vi "Data Acq Text Out.vi"(1 "Data Acq":T2={"New/Stop File"=enum."New File", "Comments Option"=FALSE, "Comments"="", "extra wait"=1} {"extra wait" min=0}) -> (0 "Command text":string[][](array[string]))   [LabVIEW 2024]
uses:
  Data Acq.ctl
panel:
  out "New/Stop File":T1(ring)
  out "String Cluster":T3
  # "AND wait extra"
  # "seconds"
  # "Advanced Control"
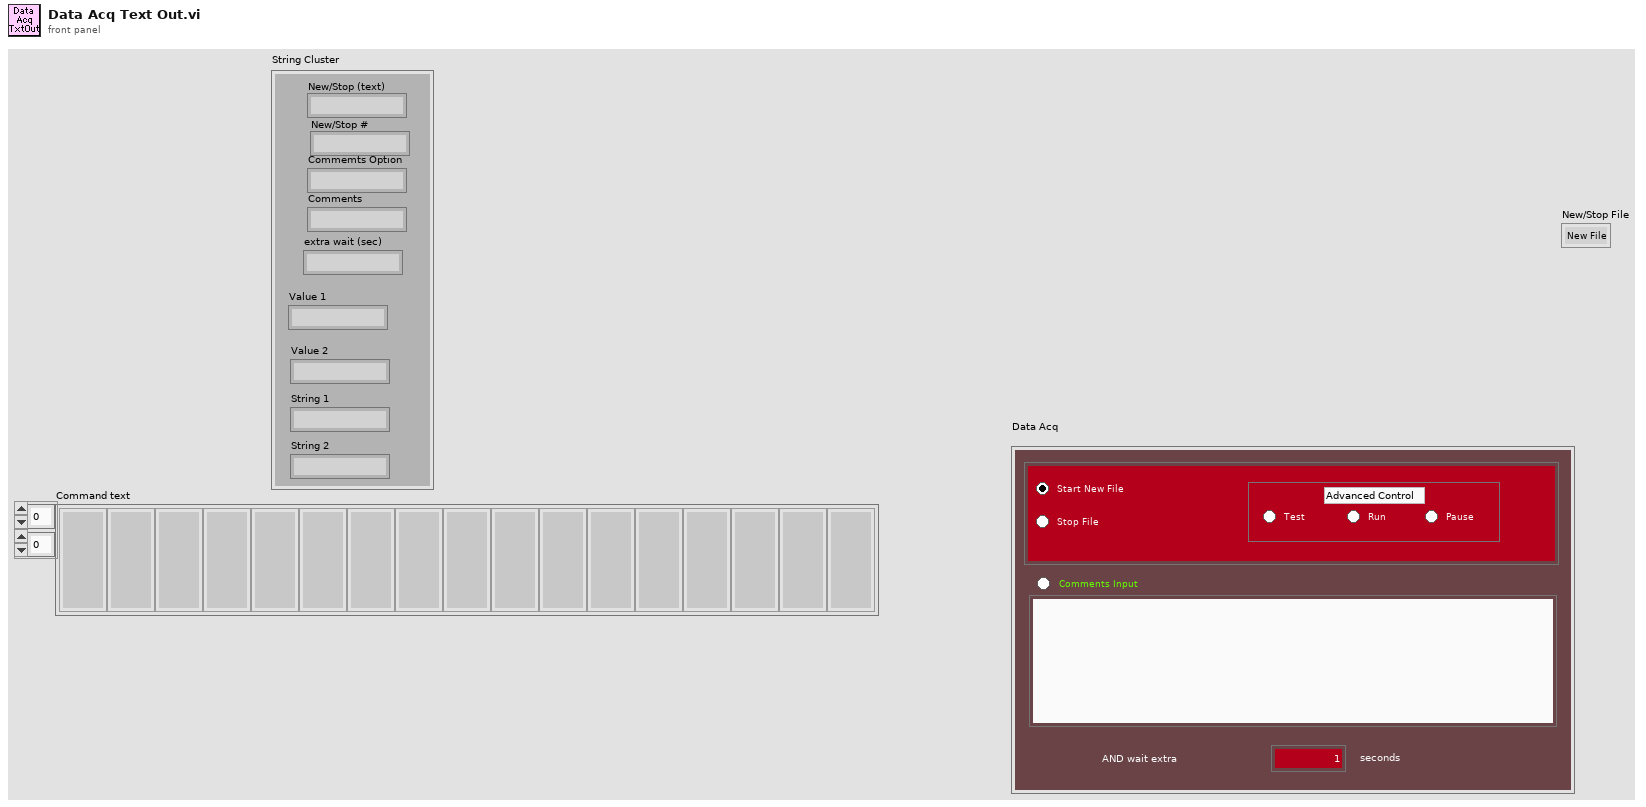
[diagram p1: front panel]
types:
  T1 = enum32{"New File", "Stop FIle", "Test", "Run", "Pause"}
  T2 = typedef "Data Acq.ctl" = cluster{"New/Stop File":enum32{"New File", "Stop FIle", "Test", "Run", "Pause"}, "Comments Option":bool, "Comments":string, "extra wait":i32}
  T3 = cluster{"New/Stop (text)":string, "Commemts Option":string, "Comments":string, "extra wait (sec)":string, "New/Stop #":string, "Value 1":string, "Value 2":string, "String 1":string, "String 2":string}
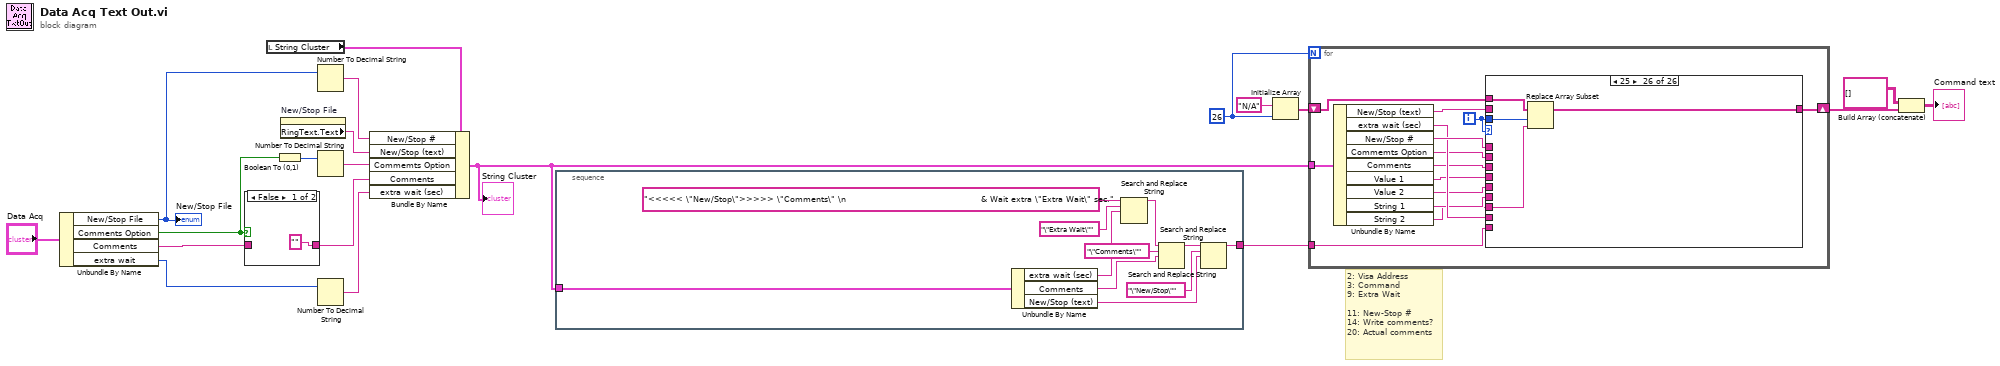
[diagram p0: block diagram]
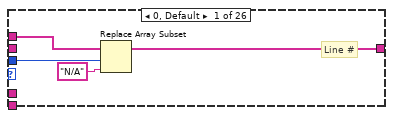
[diagram p3: hidden frame]
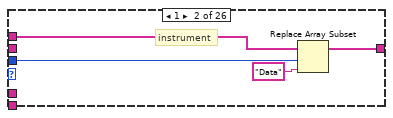
[diagram p4: hidden frame]
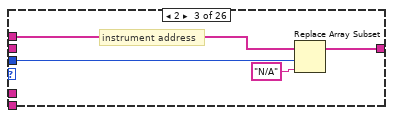
[diagram p5: hidden frame]
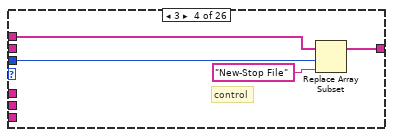
[diagram p6: hidden frame]
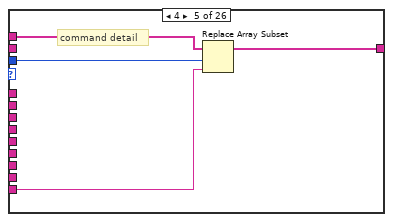
[diagram p7: hidden frame]
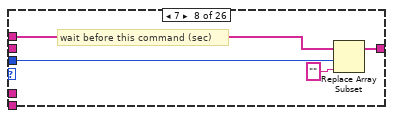
[diagram p10: hidden frame]
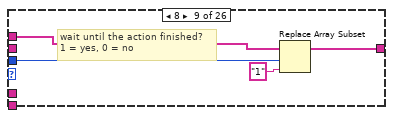
[diagram p11: hidden frame]
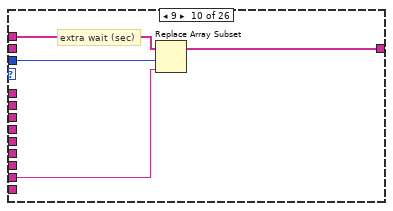
[diagram p12: hidden frame]
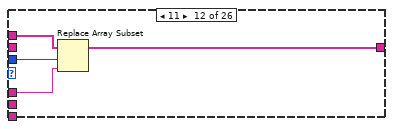
[diagram p14: hidden frame]
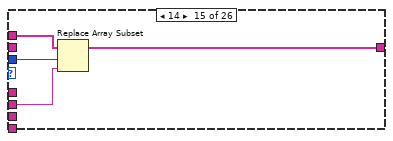
[diagram p17: hidden frame]
diagram:
  w17 = 26
  # "2: Visa Address\n3: Command\n9: Extra Wait\n\n11: New-Stop #\n14: Write comments?\n20: Actual comments"
  n1 = Unbundle By Name("Data Acq") -> ("New/Stop File"=w4:T1, "Comments Option"=w7:bool, "Comments"=w9:string, "extra wait"=w2:i32)
  "New/Stop File" <- w4
  n2 = case shown="False" w7 {
    tunnel: w9 -> [_ w22]
    tunnel: ["" w22] -> w8
    frame False {
    }
    frame True {
    }
  }
  n3 = local read "String Cluster"() -> (w14:T3)
  n4 = Boolean To (0,1)(Boolean=w7) -> (0, 1=w6:i16)
  n5 = property on="New/Stop File" class="Enum (strict)"() -> ("RingText.Text"=w10:string)  [unwired: 2 in, 2 out]
  n6 = Number To Decimal String(number=w4) -> (decimal integer string=w3:string)  [unwired: 1 in]
  n7 = Number To Decimal String(number=w6) -> (decimal integer string=w5:string)  [unwired: 1 in]
  n8 = Number To Decimal String(number=w2) -> (decimal integer string=w1:string)  [unwired: 1 in]
  n9 = Bundle By Name(cluster=w14, "New/Stop #"=w3, "New/Stop (text)"=w10, "Commemts Option"=w5, "Comments"=w8, "extra wait (sec)"=w1) -> (w12:T3)
  "String Cluster" <- w12
  n10 = stacked-sequence {
    tunnel: [w23] -> w13
    tunnel: w12 -> [w27]
    frame #0 {
      n11 = Unbundle By Name(w27) -> ("extra wait (sec)"=w26:string, "Comments"=w25:string, "New/Stop (text)"=w24:string)
      n12 = Search and Replace String(input string="<<<<< \"New/Stop\">>>>> \"Comments\" \n                                             & Wait extra \"Extra Wait\" sec.", search string="\"Extra Wait\"", replace string=w26) -> (result string=w32:string)  [unwired: 5 in, 3 out]
      n13 = Search and Replace String(input string=w32, search string="\"Comments\"", replace string=w25) -> (result string=w33:string)  [unwired: 5 in, 3 out]
      n14 = Search and Replace String(input string=w33, search string="\"New/Stop\"", replace string=w24) -> (result string=w23:string)  [unwired: 5 in, 3 out]
    }
  }
  n15 = Initialize Array("N/A", w17) -> (w16:string[])
  n16 = for {
    N: w17 -> [_]
    shift-right: [w45] -> w15
    shift-left: w16 -> [w46]
    tunnel: w13 -> [w44]
    tunnel: w12 -> [w43]
    i -> [w47]
    n17 = Unbundle By Name(w43) -> ("New/Stop (text)"=w41:string, "extra wait (sec)"=w40:string, "New/Stop #"=w42:string, "Commemts Option"=w39:string, "Comments"=w38:string, "Value 1"=w37:string, "Value 2"=w36:string, "String 1"=w35:string, "String 2"=w34:string)
    n18 = case shown="25" w47 {
      tunnel: w47 -> [w50 w54 w59 w61 w66 _ _ w71 w75 w79 _ w84 _ _ w90 _ _ _ _ _ w99 _ w103 w108 w112 w116]
      tunnel: w46 -> [w51 w53 w58 w62 w67 w68 w69 w73 w77 w81 w82 w85 w87 w88 w92 w93 w94 w95 w96 w97 w101 w102 w105 w110 w114 w117]
      tunnel: [w48 w52 w57 w60 w65 w68 w69 w72 w76 w80 w82 w86 w87 w88 w91 w93 w94 w95 w96 w97 w100 w102 w104 w109 w113 w118] -> w45
      tunnel: w44 -> [_ _ _ _ w64 _ _ _ _ _ _ _ _ _ _ _ _ _ _ _ _ _ _ _ _ _]
      tunnel: w42 -> [_ _ _ _ _ _ _ _ _ _ _ w83 _ _ _ _ _ _ _ _ _ _ _ _ _ _]
      tunnel: w41 -> [_ _ _ _ _ _ _ _ _ _ _ _ _ _ _ _ _ _ _ _ _ _ _ _ _ _]
      tunnel: w40 -> [_ _ _ _ _ _ _ _ _ w78 _ _ _ _ _ _ _ _ _ _ _ _ _ _ _ _]
      tunnel: w39 -> [_ _ _ _ _ _ _ _ _ _ _ _ _ _ w89 _ _ _ _ _ _ _ _ _ _ _]
      tunnel: w38 -> [_ _ _ _ _ _ _ _ _ _ _ _ _ _ _ _ _ _ _ _ w98 _ _ _ _ _]
      tunnel: w37 -> [_ _ _ _ _ _ _ _ _ _ _ _ _ _ _ _ _ _ _ _ _ _ w106 _ _ _]
      tunnel: w36 -> [_ _ _ _ _ _ _ _ _ _ _ _ _ _ _ _ _ _ _ _ _ _ _ w107 _ _]
      tunnel: w35 -> [_ _ _ _ _ _ _ _ _ _ _ _ _ _ _ _ _ _ _ _ _ _ _ _ w111 _]
      tunnel: w34 -> [_ _ _ _ _ _ _ _ _ _ _ _ _ _ _ _ _ _ _ _ _ _ _ _ _ w115]
      frame 0, Default {
        # "Line #"
        n19 = Replace Array Subset(array=w51, new element="N/A", index=w50) -> (w48:string[])
      }
      frame 1 {
        # "instrument"
        n20 = Replace Array Subset(array=w53, new element="Data", index=w54) -> (w52:string[])
      }
      frame 2 {
        # "instrument address"
        n21 = Replace Array Subset(array=w58, new element="N/A" ("new element/subarray"), index=w59) -> (w57:string[])
      }
      frame 3 {
        # "control"
        n22 = Replace Array Subset(array=w62, new element="New-Stop File", index=w61) -> (w60:string[])
      }
      frame 4 {
        # "command detail"
        n23 = Replace Array Subset(array=w67, new element=w64, index=w66) -> (w65:string[])
      }
      frame 5 {
        # "in  case 1"
      }
      frame 6 {
        # "in case 2"
      }
      frame 7 {
        # "wait before this command (sec)"
        n24 = Replace Array Subset(array=w73, new element="" ("new element/subarray"), index=w71) -> (w72:string[])
      }
      frame 8 {
        # "wait until the action finished?\n1 = yes, 0 = no"
        n25 = Replace Array Subset(array=w77, new element="1", index=w75) -> (w76:string[])
      }
      frame 9 {
        # "extra wait (sec)"
        n26 = Replace Array Subset(array=w81, new element=w78, index=w79) -> (w80:string[])
      }
      frame 10 {
      }
      frame 11 {
        n27 = Replace Array Subset(array=w85, new element=w83, index=w84) -> (w86:string[])
      }
      frame 12 {
      }
      frame 13 {
      }
      frame 14 {
        n28 = Replace Array Subset(array=w92, new element=w89, index=w90) -> (w91:string[])
      }
      frame 15 {
      }
      frame 16 {
      }
      frame 17 {
      }
      frame 18 {
      }
      frame 19 {
      }
      frame 20 {
        n29 = Replace Array Subset(array=w101, new element=w98, index=w99) -> (w100:string[])
      }
      frame 21 {
      }
      frame 22 {
        n30 = Replace Array Subset(array=w105, new element=w106, index=w103) -> (w104:string[])
      }
      frame 23 {
        n31 = Replace Array Subset(array=w110, new element=w107, index=w108) -> (w109:string[])
      }
      frame 24 {
        n32 = Replace Array Subset(array=w114, new element=w111, index=w112) -> (w113:string[])
      }
      frame 25 {
        n33 = Replace Array Subset(array=w117, new element=w115, index=w116) -> (w118:string[])
      }
    }
  }
  n34 = Build Array (concatenate)(string[][] [], w15) -> (→"Command text":string[][])
